vi "Sort 2D Array.vi"(5 "Order":enum16{"Ascending", "Descending"}(ring)=enum."Descending", 6 "Sort column #":i32, 7 "Array":dbl[][](array[numeric]) format="%.2f") -> (3 "Sorted Array":dbl[][](array[numeric]) format="%.2f")   [LabVIEW 2016]
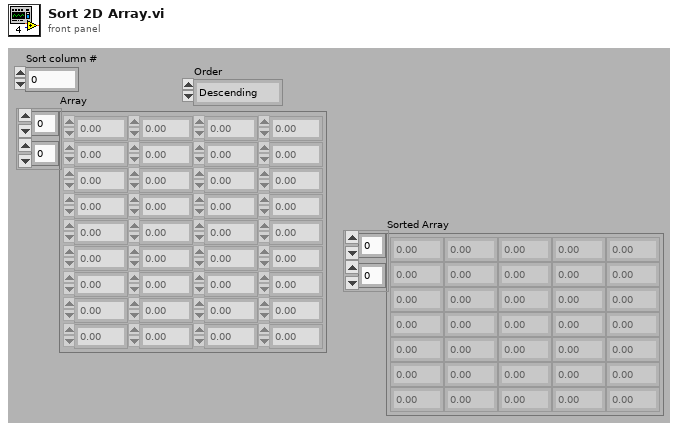
[diagram p1: front panel]
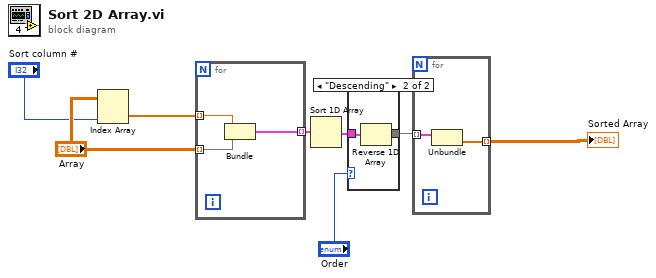
[diagram p0: block diagram]
diagram:
  n1 = Index Array(array="Array", index (col)="Sort column #") -> (element=w8:dbl[])  [unwired: 1 in]
  n2 = for {
    tunnel: "Array" -> [w11] mode=indexing
    tunnel: w8 -> [w10] mode=indexing
    tunnel: [w9] -> w7 mode=indexing
    n3 = Bundle("Numeric"=w10, "Array"=w11) -> (w9:cluster{"Numeric":dbl, "Array":dbl[]})  [unwired: 1 out]
  }
  n4 = Sort 1D Array(array=w7) -> (sorted array=w6:cluster{"Numeric":dbl, "Array":dbl[]}[])
  n5 = case shown="\"Descending\"" "Order" {
    tunnel: w6 -> [w12 w13]
    tunnel: [w12 w14] -> w4
    frame "Ascending", Default {
    }
    frame "Descending" {
      n6 = Reverse 1D Array(array=w13) -> (reversed array=w14:cluster{"Numeric":dbl, "Array":dbl[]}[])
    }
  }
  n7 = for {
    tunnel: w4 -> [w16] mode=indexing
    tunnel: [w15] -> w2 mode=indexing
    n8 = Unbundle(w16) -> ("Array"=w15:dbl[])  [unwired: 1 out]
  }
  "Sorted Array" <- w2
